vi "subDFD_Preload VIs.vi"(8 "error in (no error)":errorcluster, 10 "VI names":string[](array[string]), 11 "source folder":path) -> (0 "error out":errorcluster, 3 "all VIs refs":refnum<vi>[](array[refnum]))   [LabVIEW 2023]
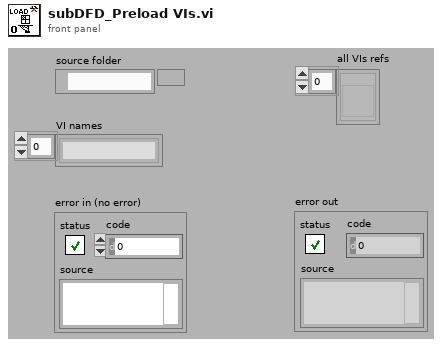
[diagram p1: front panel]
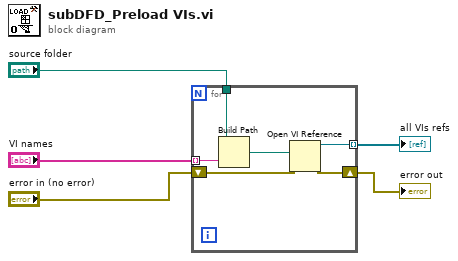
[diagram p0: block diagram]
diagram:
  n1 = for {
    tunnel: "VI names" -> [w10] mode=indexing
    tunnel: "source folder" -> [w11]
    shift-right: [w7] -> w3
    shift-left: "error in (no error)" -> [w8]
    tunnel: [w6] -> w4 mode=indexing
    n2 = Build Path(base path=w11, name or relative path=w10) -> (appended path=w9:path)
    n3 = Open VI Reference(vi path=w9, error in (no error)=w8) -> (vi reference=w6:refnum<vi>, error out=w7:errorcluster)  [unwired: 4 out]
  }
  "all VIs refs" <- w4
  "error out" <- w3
